vi "fieldshift.vi"(1 "sweep rate":dbl format="%.2f", 2 "time interval":dbl[](array[numeric]) format="%.2f", 3 "time shift":dbl format="%.2f", 4 "input field":dbl[](array[numeric]) format="%.2f") -> (0 "outut field":dbl[](array[numeric]) format="%.2f")   [LabVIEW 2018]
uses:
  <vilib>/Analysis/baseanly.llb/Mean (DBL).vi
  <vilib>/Analysis/NI_AALPro.lvlib
  <vilib>/Analysis/NI_AALBase.lvlib
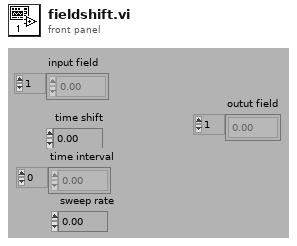
[diagram p1: front panel]
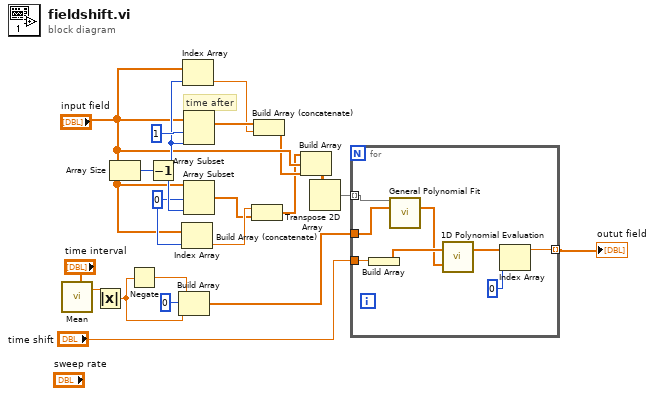
[diagram p0: block diagram]
diagram:
  w16 = 0
  # "time after"
  n1 = call-poly <vilib>:"Mean.vi"("X"="time interval") -> ("mean"=w1:dbl)  [unwired: 1 out]
  n2 = Absolute Value(x=w1) -> (abs(x)=w8:dbl)
  n3 = Array Size(array="input field") -> (size(s)=w19:i32)
  n4 = Negate(x=w8) -> (-x=w9:dbl)
  n5 = Decrement(x=w19) -> (x-1=w18:i32)
  n6 = Build Array(w9, 0, w8) -> (w6:dbl[])
  n7 = Index Array(array="input field", index=w16) -> (element=w15:dbl)
  n8 = Index Array(array="input field", index=w18) -> (element=w17:dbl)
  n9 = Array Subset(array="input field", index=1, length=w18) -> (w20:dbl[])
  n10 = Array Subset(array="input field", index=w16, length=w18) -> (w14:dbl[])
  n11 = Build Array (concatenate)(w15, w14) -> (w10:dbl[])
  n12 = Build Array (concatenate)(w20, w17) -> (w11:dbl[])
  n13 = Build Array(w10, "input field", w11) -> (w7:dbl[][])
  n14 = Transpose 2D Array(2D array=w7) -> (transposed array=w5:dbl[][])
  n15 = for {
    tunnel: w5 -> [w29] mode=indexing
    tunnel: w6 -> [w28]
    tunnel: "time shift" -> [w27]
    tunnel: [w24] -> w3 mode=indexing
    n16 = Build Array(w27) -> (w26:dbl[])
    n17 = call <vilib>:"General Polynomial Fit.vi"("Y"=w29, "X"=w28) -> ("Polynomial Coefficients"=w25:dbl[])  [unwired: 10 in, 3 out]
    n18 = call <vilib>:"1D Polynomial Evaluation.vi"("Coefficients: a"=w25, "X"=w26) -> ("Y"=w23:dbl[])  [unwired: 1 out]
    n19 = Index Array(array=w23, index=0) -> (element=w24:dbl)
  }
  "outut field" <- w3
